vi "NIIE_Mouse Down.vi"(8 "Error":errorcluster, 10 "Double Click":bool, 11 "Data":T1={"Class"={"Ants"=refnum, "Layer"=refnum, "Templates"=refnum, "Icon"=refnum, "Glyph"=refnum, "Settings"=refnum, "Tools"=refnum}, "Ref"={"Add Layer"=refnum, "Remove Layer"=refnum, "Line Text"=[], "Body Text Spec"=refnum, "DNL_Font"=refnum, "glyph path str"=refnum, "templates path str"=refnum, "Arrow Up"=refnum, "Arrow Down"=refnum, "IE VI Ref"=refnum, "Glyphs tree"=refnum, "Templates tree"=refnum, "Layer Icon Text"=refnum, "Layer Template"=refnum, "Clipboard"=refnum, "BW icon in"=refnum, "Color icon in"=refnum, "Layer Clust"=refnum, "Body Text"=refnum, "DNL_Framework Templates"=refnum, "Search Templates"=refnum, "TextMarker"=refnum, "Tab Control"=refnum, "Search Glyphs"=refnum, "Line Color"=refnum, "DNL_Glyphs []"=refnum, "Fill Color"=refnum, "Tools"=refnum, "Glyphs tree"=refnum, "Icon"=refnum, "Preview"=refnum, "Ants"=refnum, "Terminals"=refnum, "menu reference"=refnum, "LayerNames"=[], "GlyphLoadAnimation"=refnum, "TemplateLoadAnimation"=refnum, "refreshGlyphs"=refnum, "refreshTemplates"=refnum}, "Support"={"AntsRect"={"left"=0, "top"=0, "right"=0, "bottom"=0}, "Mouse Move Coords"={"Horizontal"=0, "Vertical"=0}, "Mouse Down Coords"={"Horizontal"=0, "Vertical"=0}, "Temp Coord"={"Horizontal"=0, "Vertical"=0}, "Action"=enum."Default", "Edge Color"=4914962, "Fill Color"=16860, "Mouse Down?"=FALSE, "Draft Mode?"=FALSE, "Temp Icon"=bytes[3102], "CTRL Pressed"=FALSE, "Move Selection?"=FALSE, "AntsRect Orig"={"left"=0, "top"=0, "right"=0, "bottom"=0}, "Text"="", "TM Set?"=FALSE, "Mouse inside icon?"=FALSE, "Tool (old value)"=0, "Pencil Move Color"=0, "Swap Colors?"=FALSE, "Shift pressed?"=FALSE}}) -> (0 "Error Out":errorcluster, 3 "Data Out":T1={"Class"={"Ants"=refnum, "Layer"=refnum, "Templates"=refnum, "Icon"=refnum, "Glyph"=refnum, "Settings"=refnum, "Tools"=refnum}, "Ref"={"Add Layer"=refnum, "Remove Layer"=refnum, "Line Text"=[], "Body Text Spec"=refnum, "DNL_Font"=refnum, "glyph path str"=refnum, "templates path str"=refnum, "Arrow Up"=refnum, "Arrow Down"=refnum, "IE VI Ref"=refnum, "Glyphs tree"=refnum, "Templates tree"=refnum, "Layer Icon Text"=refnum, "Layer Template"=refnum, "Clipboard"=refnum, "BW icon in"=refnum, "Color icon in"=refnum, "Layer Clust"=refnum, "Body Text"=refnum, "DNL_Framework Templates"=refnum, "Search Templates"=refnum, "TextMarker"=refnum, "Tab Control"=refnum, "Search Glyphs"=refnum, "Line Color"=refnum, "DNL_Glyphs []"=refnum, "Fill Color"=refnum, "Tools"=refnum, "Glyphs tree"=refnum, "Icon"=refnum, "Preview"=refnum, "Ants"=refnum, "Terminals"=refnum, "menu reference"=refnum, "LayerNames"=[], "GlyphLoadAnimation"=refnum, "TemplateLoadAnimation"=refnum, "refreshGlyphs"=refnum, "refreshTemplates"=refnum}, "Support"={"AntsRect"={"left"=0, "top"=0, "right"=0, "bottom"=0}, "Mouse Move Coords"={"Horizontal"=0, "Vertical"=0}, "Mouse Down Coords"={"Horizontal"=0, "Vertical"=0}, "Temp Coord"={"Horizontal"=0, "Vertical"=0}, "Action"=enum."Default", "Edge Color"=4914962, "Fill Color"=16860, "Mouse Down?"=FALSE, "Draft Mode?"=FALSE, "Temp Icon"=bytes[3102], "CTRL Pressed"=FALSE, "Move Selection?"=FALSE, "AntsRect Orig"={"left"=0, "top"=0, "right"=0, "bottom"=0}, "Text"="", "TM Set?"=FALSE, "Mouse inside icon?"=FALSE, "Tool (old value)"=0, "Pencil Move Color"=0, "Swap Colors?"=FALSE, "Shift pressed?"=FALSE}})   [LabVIEW 2021]
uses:
  Controls/IE Data.ctl
  Class/Ants/Ants.lvclass
  Class/FakedArray/FakedArray.lvclass
  Class/Icon Library/Glyph.lvclass
  Class/Settings/Settings.lvclass
  Class/Tools/Tools Paint.lvclass
  vi.lib/LabVIEW Icon API/lv_icon/Classes/Icon/Icon.lvclass
  Controls/IE Classes.ctl
  Controls/References Cluster.ctl
  Controls/SupportClass.ctl
  <vilib>/Utility/miscctls.llb/LVPoint32TypeDef.ctl
  Controls/ENUM_SupportClass_Action.ctl
  vi.lib/LabVIEW Icon API/lv_icon/Controls/IEColor.ctl
  vi.lib/LabVIEW Icon API/lv_icon/Controls/LayerType.ctl
  vi.lib/LabVIEW Icon API/lv_icon/Classes/Layer/Layer.lvclass
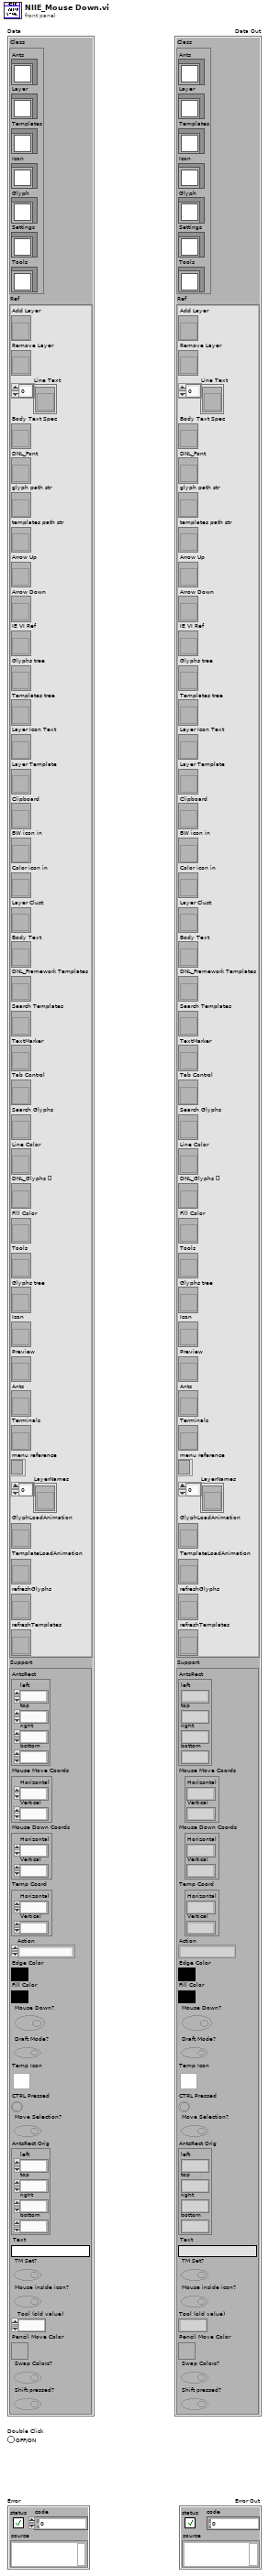
[diagram p1: front panel]
types:
  T1 = typedef "IE Data.ctl" = cluster{"Class":T2, "Ref":T3, "Support":T4}
  T2 = typedef "IE Classes.ctl" = cluster{"Ants":refnum<class "Ants.lvclass">, "Layer":refnum<class "FakedArray.lvclass">, "Templates":refnum<class "FakedArray.lvclass">, "Icon":refnum<class "Icon.lvclass">, "Glyph":refnum<class "Glyph.lvclass">, "Settings":refnum<class "Settings.lvclass">, "Tools":refnum<class "Tools Paint.lvclass">}
  T3 = typedef "References Cluster.ctl" = cluster{"Add Layer":refnum<vi>, "Remove Layer":refnum<vi>, "Line Text":refnum<vi>[], "Body Text Spec":refnum<vi>, "DNL_Font":refnum<vi>, "glyph path str":refnum<vi>, "templates path str":refnum<vi>, "Arrow Up":refnum<vi>, "Arrow Down":refnum<vi>, "IE VI Ref":refnum<vi>, "Glyphs tree":refnum<vi>, "Templates tree":refnum<vi>, "Layer Icon Text":refnum<vi>, "Layer Template":refnum<vi>, "Clipboard":refnum<vi>, "BW icon in":refnum<vi>, "Color icon in":refnum<vi>, "Layer Clust":refnum<vi>, "Body Text":refnum<vi>, "DNL_Framework Templates":refnum<vi>, "Search Templates":refnum<vi>, "TextMarker":refnum<vi>, "Tab Control":refnum<vi>, "Search Glyphs":refnum<vi>, "Line Color":refnum<vi>, "DNL_Glyphs []":refnum<vi>, "Fill Color":refnum<vi>, "Tools":refnum<vi>, "Glyphs tree":refnum<vi>, "Icon":refnum<vi>, "Preview":refnum<vi>, "Ants":refnum<vi>, "Terminals":refnum<vi>, "menu reference":refnum<k9>, "LayerNames":refnum<vi>[], "GlyphLoadAnimation":refnum<vi>, "TemplateLoadAnimation":refnum<vi>, "refreshGlyphs":refnum<vi>, "refreshTemplates":refnum<vi>}
  T4 = typedef "SupportClass.ctl" = cluster{"AntsRect":cluster{"left":i16, "top":i16, "right":i16, "bottom":i16}, "Mouse Move Coords":T5, "Mouse Down Coords":T5, "Temp Coord":T5, "Action":T6, "Edge Color":T7, "Fill Color":T7, "Mouse Down?":bool, "Draft Mode?":bool, "Temp Icon":picture, "CTRL Pressed":bool, "Move Selection?":bool, "AntsRect Orig":cluster{"left":i16, "top":i16, "right":i16, "bottom":i16}, "Text":string, "TM Set?":bool, "Mouse inside icon?":bool, "Tool (old value)":u32, "Pencil Move Color":u32, "Swap Colors?":bool, "Shift pressed?":bool}
  T5 = typedef "LVPoint32TypeDef.ctl" = cluster{"Horizontal":i32, "Vertical":i32}
  T6 = typedef "ENUM_SupportClass_Action.ctl" = enum16{"Default", "Move Selection", "Glyph Library", "Tool"}
  T7 = typedef "IEColor.ctl" = u32
  T8 = typedef "LayerType.ctl" = enum16{"Graphic", "Text", "Tool", "Graphic Drop"}
  T9 = cluster{"left":i16, "top":i16, "right":i16, "bottom":i16}
  T10 = typedef "Cluster_Button Draw Tools.ctl" = enum32{"Pencil", "Line", "Dropper", "Fill", "Rectangle", "Filled Rectangle", "Ellipse", "Filled Ellipse", "Eraser", "Text", "Select", "Move"}
  T11 = typedef "Cluster_INI Data.ctl" = cluster{"Show Layer Tab?":bool, "Show Terminals?":bool, "Text":cluster{"Font":T12, "Alignment":T13, "Size":T14}, "3rd party Templates":cluster{"Store 3rd party Templates?":bool, "Folder Name":string}, "Merge user layers on commit":bool, "Body Text":T15, "Fill Color":T7, "Edge Color":T7, "Tab":u16, "Tool":T10, "Disable Layers?":bool}
  T12 = typedef "Font.ctl" = string
  T13 = typedef "Alignment.ctl" = u16
  T14 = typedef "Num_Font Size.ctl" = u8
  T15 = typedef "Cluster_BodyText.ctl" = cluster{"Line 1 text":string, "Line 2 text":string, "Line 3 text":string, "Line 4 text":string, "Line 1 color":u32, "Line 2 color":u32, "Line 3 color":u32, "Line 4 color":u32, "Body Text Spec":cluster{"Font":T12, "Alignment":T13, "Size":u8}, "Center text vertically":bool, "Capitalize Text":bool}
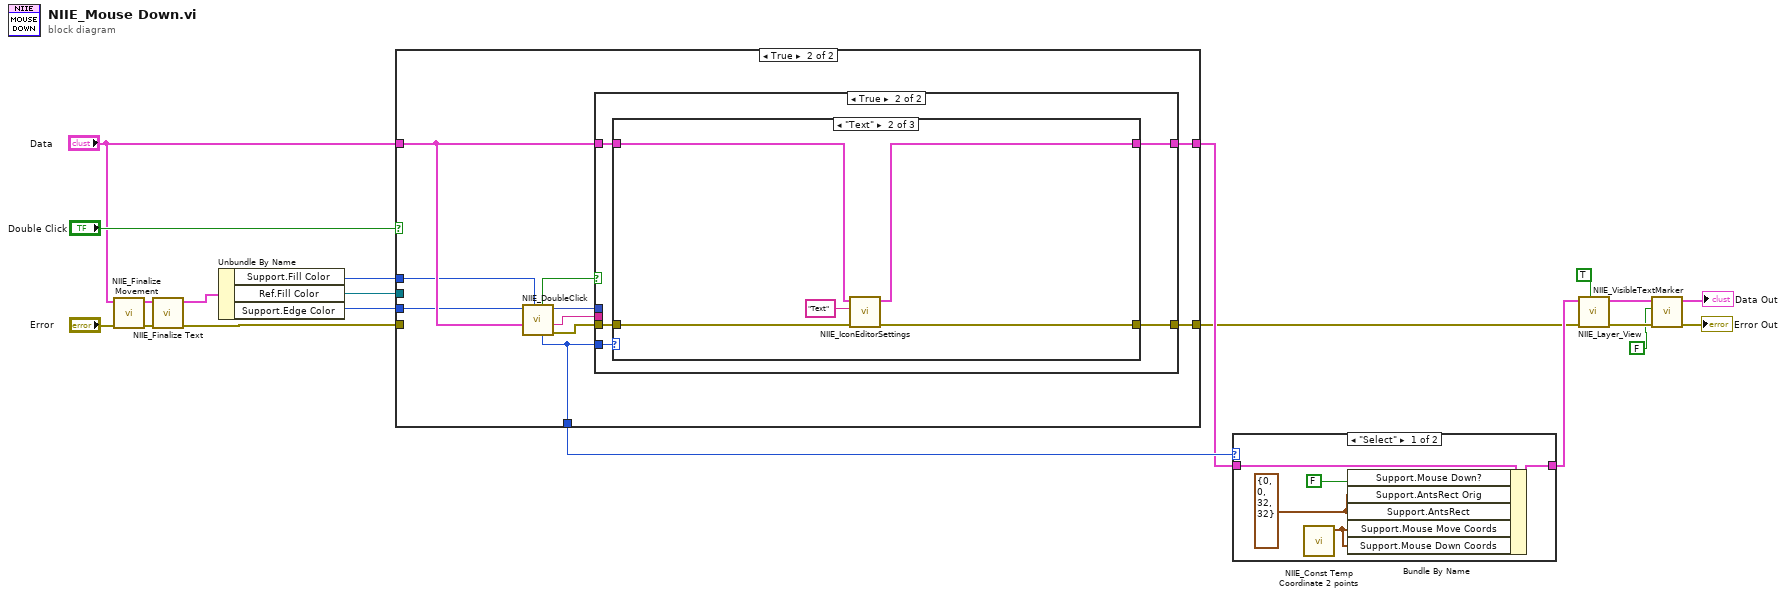
[diagram p0: block diagram]
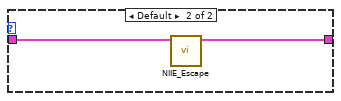
[diagram p2: hidden frame]
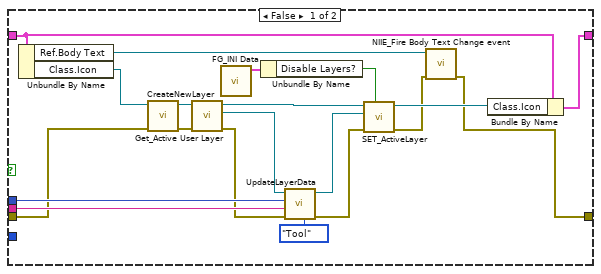
[diagram p4: hidden frame]
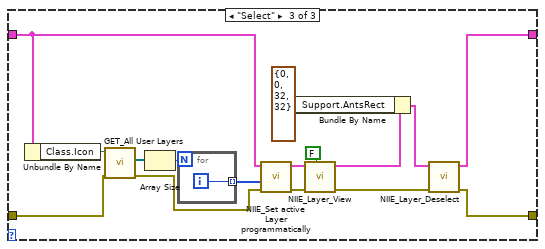
[diagram p6: hidden frame]
diagram:
  n1 = call "NIIE_Finalize Movement.vi"("Error"="Error", "Data"="Data") -> ("Error Out"=w13:errorcluster, "Data Out"=w11:T1)  [unwired: 1 in, 7 out]
  n2 = call "NIIE_Finalize Text.vi"("Error"=w13, "Data"=w11) -> ("Error Out"=w9:errorcluster, "Data Out"=w10:T1)  [unwired: 8 out]
  n3 = Unbundle By Name(w10) -> ("Support.Fill Color"=w1:T7, "Ref.Fill Color"=w17:refnum<vi>, "Support.Edge Color"=w19:T7)
  n4 = case shown="True" "Double Click" {
    tunnel: w9 -> [w22 _]
    tunnel: w19 -> [_ w23]
    tunnel: [w22 w31] -> w2
    tunnel: [_ w28] -> w20
    tunnel: w17 -> [_ _]
    tunnel: "Data" -> [w21 w27]
    tunnel: [w21 w26] -> w3
    tunnel: w1 -> [_ w25]
    frame False {
    }
    frame True {
      n5 = call "NIIE_DoubleClick.vi"("Fill Color"=w25, "Data"=w27, "Edge Color"=w23) -> ("Error Out"=w32:errorcluster, "Name Out"=w30:string, "New Picture Out"=w24:picture, "Active Tool Out"=w28:T10, "Invalid Picture? Out"=w29:bool)  [unwired: 2 in, 2 out]
      n6 = case shown="True" w29 {
        tunnel: w32 -> [w49 w56]
        tunnel: [w36 w55] -> w31
        tunnel: w24 -> [w52 _]
        tunnel: w30 -> [w51 _]
        tunnel: w28 -> [_ w57]
        tunnel: w27 -> [w38 w54]
        tunnel: [w50 w53] -> w26
        frame False {
          n7 = Unbundle By Name(w38) -> ("Ref.Body Text"=w35:refnum<vi>, "Class.Icon"=w40:refnum<class "Icon.lvclass">)
          n8 = call "CreateNewLayer.vi"("error in"=w49, "Icon.lvclass"=w40) -> ("error out"=w48:errorcluster, "Icon.lvclass out"=w47:refnum<class "Icon.lvclass">)  [unwired: 3 in, 5 out]
          n9 = call-dynamic "Get_Active User Layer.vi"("error in (no error)"=w48, "Icon in"=w47) -> ("error out"=w45:errorcluster, "Layer.lvclass"=w44:refnum<class "Layer.lvclass">, "Icon out"=w46:refnum<class "Icon.lvclass">)  [unwired: 7 out]
          n10 = call "FG_INI Data.vi"() -> ("INI Data Out"=w34:T11)  [unwired: 9 in, 2 out]
          n11 = Unbundle By Name(w34) -> ("Disable Layers?"=w33:bool)
          n12 = call "UpdateLayerData.vi"("Type"=LayerType."Tool", "error in"=w45, "LayerName"=w51, "new picture"=w52, "Active Layer"=w44) -> ("error out"=w42:errorcluster, "Layer.lvclass out"=w43:refnum<class "Layer.lvclass">)  [unwired: 3 in, 2 out]
          n13 = call-dynamic "SET_ActiveLayer.vi"("Combine User Layers?"=w33, "Error"=w42, "Layer.lvclass"=w43, "Icon.lvclass"=w46) -> ("Error Out"=w37:errorcluster, "Icon.lvclass Out"=w39:refnum<class "Icon.lvclass">)  [unwired: 6 out]
          n14 = call "NIIE_Fire Body Text Change event.vi"("error in"=w37, "Ref.Body Text"=w35) -> ("error out"=w36:errorcluster)  [unwired: 2 in, 7 out]
          n15 = Bundle By Name(cluster=w38, "Class.Icon"=w39) -> (w50:T1)
        }
        frame True {
          n16 = case shown="\"Text\"" w57 {
            tunnel: w56 -> [w59 w64 w72]
            tunnel: [w59 w61 w65] -> w55
            tunnel: w54 -> [w58 w62 w71]
            tunnel: [w58 w60 w66] -> w53
            frame "Ellipse", Default {
            }
            frame "Text" {
              n17 = call "NIIE_IconEditorSettings.vi"("error in (no error)"=w64, "Active Tag"="Text", "Data in"=w62) -> ("error out"=w61:errorcluster, "Data out"=w60:T1)  [unwired: 7 out]
            }
            frame "Select" {
              n18 = Unbundle By Name(w71) -> ("Class.Icon"=w70:refnum<class "Icon.lvclass">)
              n19 = call-dynamic "GET_All User Layers.vi"("error in (no error)"=w72, "Icon.lvclass in"=w70) -> ("error out"=w77:errorcluster, "User Layer"=w80:refnum<class "Layer.lvclass">[])  [unwired: 7 in, 1 out]
              n20 = Array Size(array=w80) -> (size(s)=w79:i32)
              n21 = for {
                N: w79 -> [_]
                tunnel: [w81] -> w78 mode=indexing
                i -> [w81]
              }
              n22 = call "NIIE_Set active Layer programmatically.vi"("Error"=w77, "Active Layer []"=w78, "Data"=w71) -> ("Error Out"=w74:errorcluster, "Data Out"=w75:T1)  [unwired: 7 in]
              n23 = call "NIIE_Layer_View.vi"("Add To Undo?"=FALSE ("Add to Undo?"), "Error"=w74, "Data"=w75) -> ("Error Out"=w67:errorcluster, "Data Out"=w69:T1)  [unwired: 1 in, 6 out]
              n24 = Bundle By Name(cluster=w69, "Support.AntsRect"=T9 {"left"=0, "top"=0, "right"=32, "bottom"=32}) -> (w68:T1)
              n25 = call "NIIE_Layer_Deselect.vi"("Error"=w67, "Data"=w68) -> ("Error Out"=w65:errorcluster, "Data Out"=w66:T1)  [unwired: 8 out]
            }
          }
        }
      }
    }
  }
  n26 = case shown="\"Select\"" w20 {
    tunnel: w3 -> [w84 w88]
    tunnel: [w83 w87] -> w7
    frame "Select" {
      w82 = T9 {"left"=0, "top"=0, "right"=32, "bottom"=32} ("Support.AntsRect Orig")
      n27 = call "NIIE_Const Temp Coordinate 2 points.vi"() -> ("Const Temp Coordinate"=w85:T5)  [unwired: 11 out]
      n28 = Bundle By Name(cluster=w84, "Support.Mouse Down?"=FALSE ("Mouse Down?"), "Support.AntsRect Orig"=w82, "Support.AntsRect"=w82, "Support.Mouse Move Coords"=w85, "Support.Mouse Down Coords"=w85) -> (w83:T1)
    }
    frame Default {
      n29 = call "NIIE_Escape.vi"("Data"=w88) -> ("Data Out"=w87:T1)  [unwired: 2 in, 8 out]
    }
  }
  n30 = call "NIIE_Layer_View.vi"("Add To Undo?"=TRUE ("Add to Undo?"), "Error"=w2, "Data"=w7) -> ("Error Out"=w15:errorcluster, "Data Out"=w6:T1)  [unwired: 2 in, 5 out]
  n31 = call "NIIE_VisibleTextMarker.vi"("Error"=w15, "Visible"=FALSE, "Data"=w6) -> ("Error Out"=→"Error Out":errorcluster, "Data Out"=→"Data Out":T1)  [unwired: 1 in, 6 out]
